vi "Fill Uninitialized While.vi"(6 "Dimension to check":i32, 8 "Error In":errorcluster, 9 "Ref Array":dbl[](array[numeric]), 10 "Data Array Size":i32[](array[numeric])) -> (0 "Error Out":errorcluster, 1 "Ref Array out":dbl[](array[numeric]))   [LabVIEW 2017]
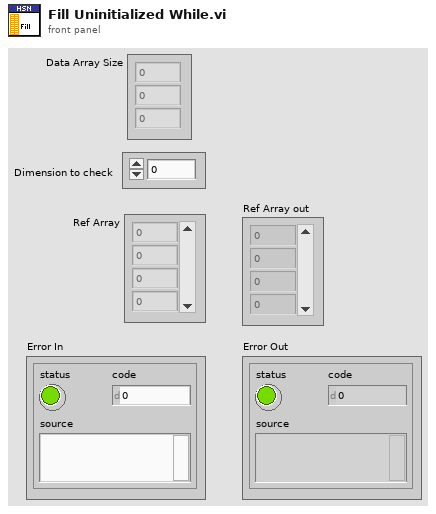
[diagram p1: front panel]
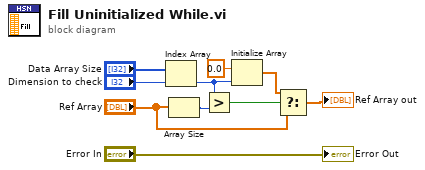
[diagram p0: block diagram]
diagram:
  n1 = Index Array(array="Data Array Size", index="Dimension to check") -> (element=w9:i32)
  n2 = Array Size(array="Ref Array") -> (size(s)=w5:i32)
  n3 = Greater?(x=w9, y=w5) -> (0:w6:bool)
  n4 = Initialize Array(0.0 ("element"), w9) -> (w10:dbl[])
  n5 = Select(t=w10, s=w6, f="Ref Array") -> (s? t:f=→"Ref Array out":dbl[])
  "Error Out" <- "Error In"
